vi "ComboBoxFromDB.vi"(8 "error in (no error)":errorcluster, 9 "connection information":path=path "e:/m100/data/m1003.dsn", 10 "Column":string, 11 "table":string) -> (0 "error out":errorcluster, 2 "Array":cluster{"String":string, "Value":string}[](array[cluster]))   [LabVIEW 2012]
uses:
  <vilib>/addons/database/Auxilliary.llb/DB Tools Cursor Type.ctl
  <vilib>/addons/database/Connection.llb/DB Tools Open Connec (Path).vi
  <vilib>/addons/database/Connection.llb/Conn Execute.vi
  <vilib>/addons/database/Recordset.llb/Rec Fetch Recordset Data (R).vi
  <vilib>/addons/database/Recordset.llb/Rec Destroy - Connection.vi
  <vilib>/addons/database/_DB Variant To Data/Database Variant To Data.xnode
  <vilib>/addons/database/NI_Database_API.lvlib
panel:
  in  "input cluster":cluster{"String":string, "Value":string}
types:
  T1 = typedef "NI_Database_API.lvlib/DB Tools Cursor Type.ctl" = enum16{"forward-only", "keyset", "dynamic", "static"}
  T2 = typedef "NI_Database_API.lvlib/Conn ObjectReference.ctl" = refnum<k1>
  T3 = typedef "NI_Database_API.lvlib/Rec ObjectReference.ctl" = refnum<k1>
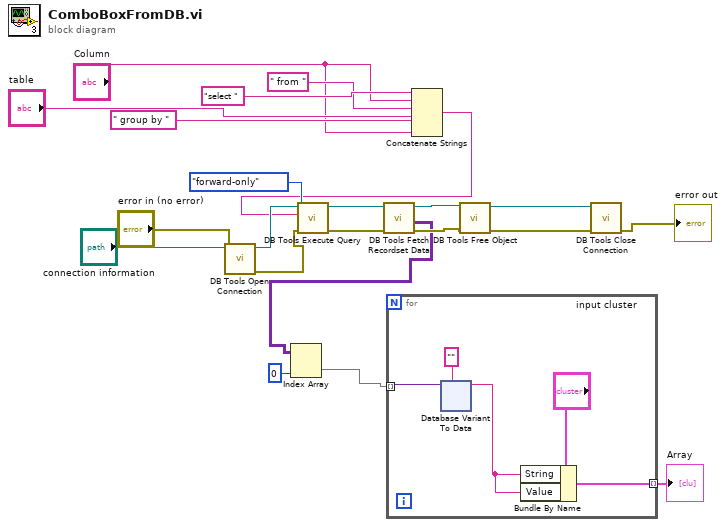
[diagram p0: block diagram]
diagram:
  n1 = call-poly <vilib>:"DB Tools Open Connection.vi"("error in (no error)"="error in (no error)", "connection information"="connection information") -> ("error out"=w19:errorcluster, "connection reference"=w20:T2)  [unwired: 6 in]
  n2 = Concatenate Strings("select " ("string"), "Column", " from " ("string"), "table", " group by " ("string"), "Column") -> (w3:string)
  n3 = call-poly <vilib>:"DB Tools Execute Query.vi"("error in (no error)"=w19, "cursor type"=DB_Tools_Cursor_Type."forward-only", "SQL query"=w3, "connection reference"=w20) -> ("error out"=w14:errorcluster, "recordset reference"=w15:T3)  [unwired: 4 in]
  n4 = call-poly <vilib>:"DB Tools Fetch Recordset Data.vi"("error in (no error)"=w14, "recordset reference"=w15) -> ("error out"=w12:errorcluster, "recordset data"=w11:variant[][], "recordset reference out"=w13:T3)  [unwired: 3 in]
  n5 = Index Array(array=w11, index (col)=0) -> (element=w10:variant[])  [unwired: 1 in]
  n6 = for {
    tunnel: w10 -> [w27] mode=indexing
    tunnel: [w23] -> w1 mode=indexing
    n7 = xnode "Database Variant To Data"("database variant"=w27, "type"="") -> ("data"=w24:string)  [unwired: 1 in, 1 out]
    n8 = Bundle By Name(cluster="input cluster", "String"=w24, "Value"=w24) -> (w23:cluster{"String":string, "Value":string})
  }
  "Array" <- w1
  n9 = call-poly <vilib>:"DB Tools Free Object.vi"("error in (no error)"=w12, "recordset reference"=w13) -> ("error out"=w17:errorcluster, "connection reference"=w18:T2)  [unwired: 8 in]
  n10 = call <vilib>:"DB Tools Close Connection.vi"("error in (no error)"=w17, "connection reference"=w18) -> ("error out"=→"error out":errorcluster)  [unwired: 5 in]
